vi "Pre Loop Init.vi"(8 "error in":errorcluster, 10 "Ref In":refnum<vi>) -> (0 "error out":errorcluster, 3 "Event Registration Refnum":refnum<event-registration>)   [LabVIEW 2018, in "Display.lvlib"]
uses:
  Display.lvlib
  User Events/controls/Actions.ctl
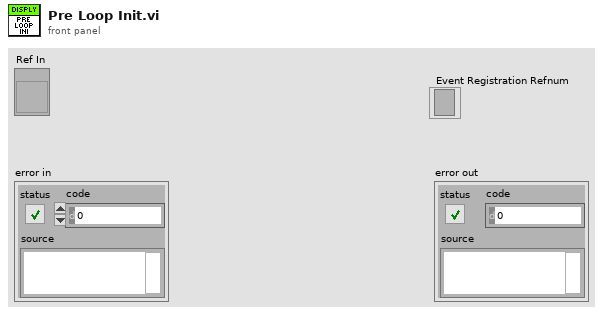
[diagram p1: front panel]
types:
  T1 = typedef "Actions.ctl" = enum16{"Get", "Create", "Destroy"}
  T2 = cluster{"Variant":variant, "action":enum16{"error", "exit", "init"}}
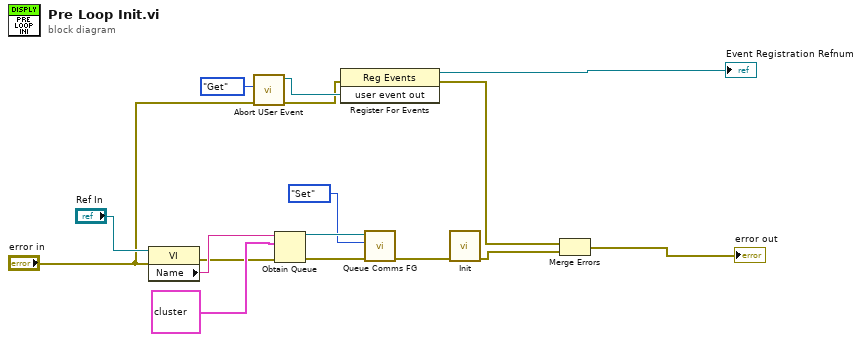
[diagram p0: block diagram]
diagram:
  n1 = property class="VI"(reference="Ref In", error in="error in") -> (error out=w7:errorcluster, "Name"=w15:string)  [unwired: 1 out]
  n2 = call "Abort USer Event.vi"("error in"="error in", "Enum"=Actions."Get") -> ("error out"=w1:errorcluster, "user event out"=w4:refnum<user-event>)  [unwired: 8 in]
  n3 = Obtain Queue(name (unnamed)=w15, element data type=T2 {"Variant"=variant, "action"=enum."init"} ("Module Data Cluster"), error in (no error)=w7) -> (queue out=w12:refnum<queue>, error out=w13:errorcluster)  [unwired: 2 in, 1 out]
  n4 = register-events(error in=w1, w4) -> (reference out=→"Event Registration Refnum":refnum<event-registration>, error out=w3:errorcluster)  [unwired: 1 in]
  n5 = call "Queue Comms FG.vi"("error in"=w13, "Action"=enum16{"Release", "Get", "Set"}."Set", "queue in"=w12) -> ("error out"=w10:errorcluster)  [unwired: 7 in, 1 out]
  n6 = call "Init.vi"("error in"=w10) -> ("error out"=w9:errorcluster)  [unwired: 10 in]
  n7 = Merge Errors(w3, w9) -> (→"error out":errorcluster)
